vi "getOpenFileNames.vi"(5 "parent":refnum<class "QWidget.lvclass">, 6 "filter":string, 8 "Error In":errorcluster, 9 "dir":string, 10 "caption":string) -> (0 "Error Out":errorcluster, 2 "Value":string[](array[string]))   [LabVIEW 2014, in "QFileDialog.lvclass"]
doc: "LabVIEW-specific documentation is not yet available. See <b>http://doc.qt.io/qt-5/QFileDialog.html#getOpenFileNames</b>"
uses:
  QFileDialog.lvclass
  QWidget/QWidget.lvclass
  LQ Core/LQIdentity/LQIdentity.lvclass/LQIdentity.ctl
  LQ Core/LQ Core.lvlib
  LQ Core/LQIdentity/LQIdentity.lvclass
panel:
  # "Copyright (c) 2016 Sze Howe Koh\n\nThis Source Code Form is subject to the terms of the Mozilla Public\nLicense, v. 2.0. If a copy of the MPL was not distributed with this\nfile, You can obtain one at http://mozilla.org/MPL/2.0/."
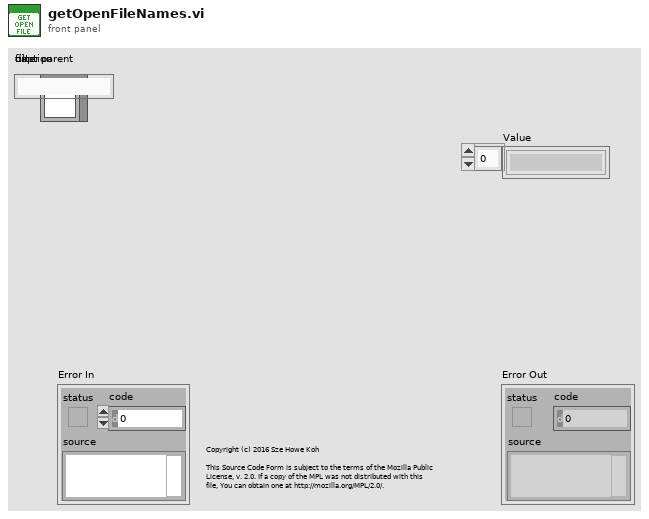
[diagram p1: front panel]
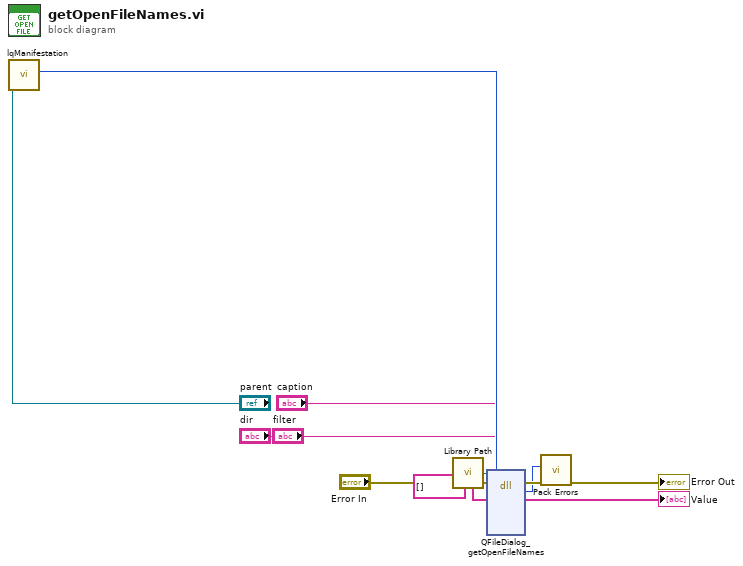
[diagram p0: block diagram]
diagram:
  n1 = call "lqManifestation.vi"("LQIdentity in"="parent") -> ("Manifestation"=w4:u64)  [unwired: 9 in, 1 out]
  n2 = call "Library Path.vi"() -> ("Library Path"=w10:path)
  n3 = dll-call lib="?" fn="QFileDialog_getOpenFileNames"(path in=w10, error in="Error In", "_retVal"=string[] [] ("retVal"), "parent"=w4, "caption"="caption", "dir"="dir", "filter"="filter") -> (error out=w8:errorcluster, w6:i32, "_retVal"=→"Value":string[])  [unwired: 5 in, 1 out]
  n4 = call "Pack Errors.vi"("Error In"=w8, "Error Code"=w6) -> ("Error Out"=→"Error Out":errorcluster)  [unwired: 9 in]
